vi "solve_for_coag(updated).vi"(4 "data":variant, 5 "x":dbl) -> (2 "f(x)":dbl)   [LabVIEW 2019]
uses:
  give_data_NR.ctl
  RowData_Type.ctl
  enum_observed_clarified.ctl
  Global Plantita Parameters.vi
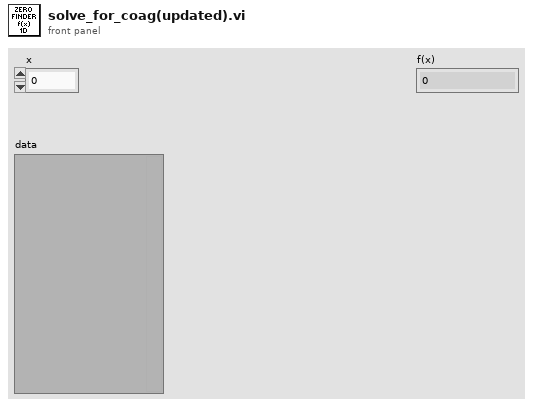
[diagram p1: front panel]
types:
  T1 = typedef "give_data_NR.ctl" = cluster{"RowData":T2, "Enum":T3}
  T2 = typedef "RowData_Type.ctl" = cluster{"C_raw(mg/L)":dbl, "C_clarified(mg/L)":dbl, "C_floc(mg/L)":dbl, "floc_sat":dbl, "C_DOM":dbl, "C_coag(mg/L)":dbl, "C_clar_target(mg/L)":dbl}
  T3 = typedef "enum_observed_clarified.ctl" = enum16{"Observed", "Target"}
  T4 = cluster{"height_ff (m)":dbl, "C_coag_stock (g/L)":dbl, "flocculation_time(min)":dbl, "clarification_time(min)":dbl, "data_interval (min)":dbl, "kpf":dbl, "kc":dbl, "q":dbl}
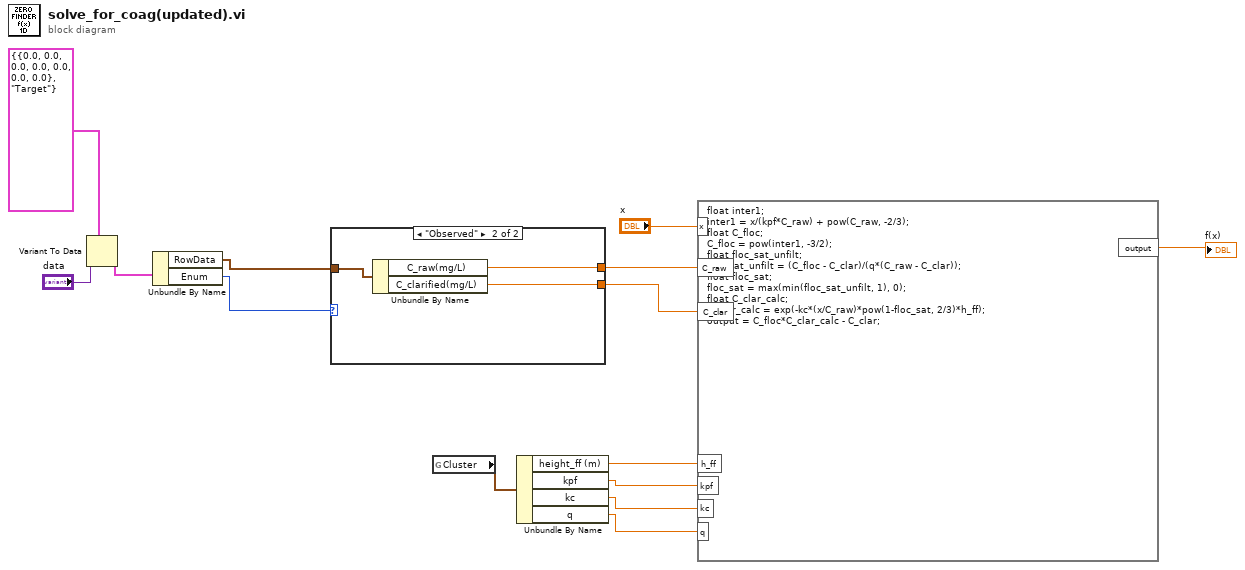
[diagram p0: block diagram]
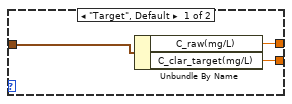
[diagram p2: hidden frame]
diagram:
  n1 = Variant To Data(type=T1 {"RowData"={"C_raw(mg/L)"=0.0, "C_clarified(mg/L)"=0.0, "C_floc(mg/L)"=0.0, "floc_sat"=0.0, "C_DOM"=0.0, "C_coag(mg/L)"=0.0, "C_clar_target(mg/L)"=0.0}, "Enum"=enum."Target"} ("data to NR"), Variant="data") -> (data=w3:T1)  [unwired: 1 in, 1 out]
  n2 = Unbundle By Name(w3) -> ("RowData"=w2:T2, "Enum"=w1:T3)
  n3 = case shown="\"Observed\"" w1 {
    tunnel: w2 -> [w17 w20]
    tunnel: [w16 w19] -> w11
    tunnel: [w15 w18] -> w10
    frame "Target", Default {
      n4 = Unbundle By Name(w17) -> ("C_raw(mg/L)"=w16:dbl, "C_clar_target(mg/L)"=w15:dbl)
    }
    frame "Observed" {
      n5 = Unbundle By Name(w20) -> ("C_raw(mg/L)"=w19:dbl, "C_clarified(mg/L)"=w18:dbl)
    }
  }
  n6 = global read "Global Plantita Parameters.vi" "Cluster"() -> (w9:T4)
  n7 = Unbundle By Name(w9) -> ("height_ff (m)"=w8:dbl, "kpf"=w7:dbl, "kc"=w6:dbl, "q"=w5:dbl)
  n8 = formula code="float inter1;\ninter1 = x/(kpf*C_raw) + pow(C_raw, -2/3);\nfloat C_floc;\nC_floc = pow(inter1, -3/2);\nfloat floc_sat_unfilt;\nfloc_sat_unfilt = (C_floc - C_clar)/(q*(C_raw - C_clar));\nfloat floc_sat;\nfloc_sat = max(min(floc_sat_unfilt, 1), 0);\nfloat C_clar_calc;\nC_clar_calc = exp(-kc*(x/C_raw)*pow(1-floc_sat, 2/3)*h_ff);\noutput = C_floc*C_clar_calc - C_clar;"("x"="x", "kpf"=w7, "C_raw"=w11, "C_clar"=w10, "kc"=w6, "h_ff"=w8, "q"=w5) -> ("output"=→"f(x)":dbl)
